vi "DFD Classical Design.vi"(5 "design method":T3(ring)=enum."Elliptic", 6 "fs [Hz]":dbl=1.0 format="%.2f", 7 "filter type":T10(ring), 8 "error in (no error)":errorcluster, 9 "ripple specs":T1={"passband"=0.1, "stopband"=60.0, "dB/linear? (T: dB)"=TRUE}, 10 "freq specs [Hz]":T2={"fpass 1"=0.2, "fstop 1"=0.3, "fpass 2 "=0.0, "fstop 2"=0.0}) -> (0 "error out":errorcluster, 2 "order":i32, 3 "filter out":T4={"mSRate_Fs"=1.0, "mSRate_Version"="2.0", "mSRate_Comments"="", "mSRate_OrgCoef"={"type"=enum."Undefined", "gain"=1.0, "coef a (k)"=[], "coef b (v)"=[]}, "mSRate_CurCoef"={"type"=enum."Undefined", "gain"=1.0, "coef a (k)"=[], "coef b (v)"=[]}, "mSRate_Quantized?"=FALSE, "mSRate_QCoef"={"type"=enum."Undefined", "gain"=1.0, "coef a (k)"=[], "coef b (v)"=[]}, "mSRate_QSettings"=[], "mSRate_Order"=0, "mSRate_Scaling"={"mSRate_ScaleByPowerOf2?"=FALSE, "mSRate_ScaleType"=enum."No Norm"}} {"mSRate_QSettings"."source" items=["Coef a/k"=0, "Coef b/v"=7, "Input"=1, "Output"=2, "Multiplicand"=3, "Product"=4, "Sum"=5, "Delay"=6, "Gain"=8]})   [LabVIEW 2017, in "NI_DigFilterLicensed.lvlib"]
doc: "Creates a lowpass, highpass, bandpass, or bandstop filter."
uses:
  <vilib>/addons/Digital Filter Design/NI_DigFilterLicensed.lvlib
  <vilib>/addons/Digital Filter Design/_Objects.llb/DFD Filter Obj.ctl
  <vilib>/addons/Digital Filter Design/_Objects.llb/DFD Filter Coef.ctl
  <vilib>/addons/Digital Filter Design/_Objects.llb/DFD Filter Structure Type Selector.ctl
  <vilib>/addons/Digital Filter Design/_Objects.llb/dfd_Internal Quantization Settings.ctl
  <vilib>/addons/Digital Filter Design/_Objects.llb/dfd_Internal Quantization Srcs.ctl
  <vilib>/addons/Digital Filter Design/_Objects.llb/DFD Coef Norm Type.ctl
  <vilib>/addons/Digital Filter Design/_Objects.llb/DFD Filter Frequence Specification (Design).ctl
  <vilib>/addons/Digital Filter Design/_Objects.llb/DFD Filter Ripple Specification (Design).ctl
  <vilib>/addons/Digital Filter Design/_REMEZ.llb/remez_fir filter type.ctl
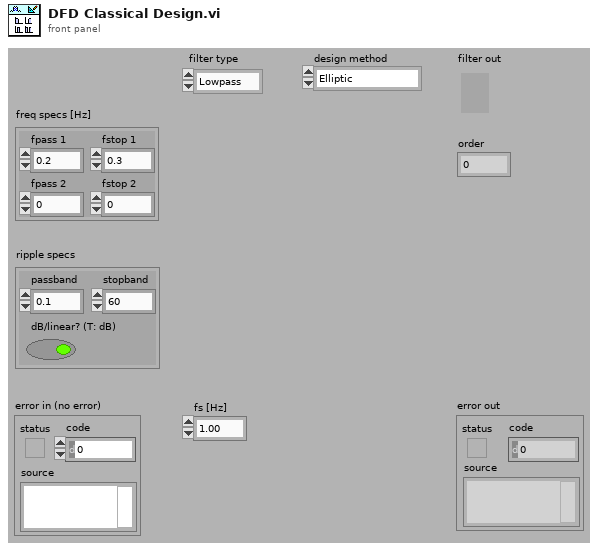
[diagram p1: front panel]
types:
  T1 = typedef "NI_DigFilterLicensed.lvlib/DFD Filter Ripple Specification (Design).ctl" = cluster{"passband":dbl, "stopband":dbl, "dB/linear? (T: dB)":bool}
  T2 = typedef "NI_DigFilterLicensed.lvlib/DFD Filter Frequence Specification (Design).ctl" = cluster{"fpass 1":dbl, "fstop 1":dbl, "fpass 2 ":dbl, "fstop 2":dbl}
  T3 = enum16{"Butterworth", "Chebyshev", "Inverse Chebyshev", "Elliptic", "Kaiser Window", "Dolph-Chebyshev Window", "Equi-Ripple FIR"}
  T4 = typedef "NI_DigFilterLicensed.lvlib/DFD Filter Obj.ctl" = cluster{"mSRate_Fs":dbl, "mSRate_Version":string, "mSRate_Comments":string, "mSRate_OrgCoef":T5, "mSRate_CurCoef":T5, "mSRate_Quantized?":bool, "mSRate_QCoef":T5, "mSRate_QSettings":T7[], "mSRate_Order":i32, "mSRate_Scaling":cluster{"mSRate_ScaleByPowerOf2?":bool, "mSRate_ScaleType":T9}}
  T5 = typedef "NI_DigFilterLicensed.lvlib/DFD Filter Coef.ctl" = cluster{"type":T6, "gain":dbl, "coef a (k)":dbl[], "coef b (v)":dbl[]}
  T6 = typedef "NI_DigFilterLicensed.lvlib/DFD Filter Structure Type Selector.ctl" = enum16{"Undefined", "FIR Direct Form", "FIR Direct Form Transposed", "FIR Symmetric", "FIR Antisymmetric", "IIR Direct Form I", "IIR Direct Form I Transposed", "IIR Direct Form II", "IIR Direct Form II Transposed", "IIR Cascaded Second Order Sections Form I", "IIR Cascaded Second Order Sections Form I Transposed", "IIR Cascaded Second Order Sections Form II", "IIR Cascaded Second Order Sections Form II Transposed", "Lattice Allpass (basic sections)", "Lattice Allpass (one multiplier sections)", "Lattice Allpass (normalized sections)", "Lattice AR (basic sections)", "Lattice AR (one multiplier sections)", "Lattice AR (normalized sections)", "Lattice MA (minimum phase)", "Lattice MA (maximum phase)", "Lattice ARMA (basic sections)", "Lattice ARMA (one multiplier sections)", "Lattice ARMA (normalized sections)"}
  T7 = typedef "NI_DigFilterLicensed.lvlib/dfd_Internal Quantization Settings.ctl" = cluster{"source":T8, "wl":i16, "iwl":i16, "overflow mode":enum16{"Saturation", "Wrap"}, "rounding mode":enum16{"Nearest", "Truncation"}, "signed?":bool}
  T8 = typedef "NI_DigFilterLicensed.lvlib/dfd_Internal Quantization Srcs.ctl" = u16
  T9 = typedef "NI_DigFilterLicensed.lvlib/DFD Coef Norm Type.ctl" = enum16{"No Norm", "Time Domain 1-Norm", "Time Domain 2-Norm", "Time Domain Inf-Norm"}
  T10 = enum16{"Lowpass", "Highpass", "Bandpass", "Bandstop"}
  T11 = typedef "NI_DigFilterLicensed.lvlib/remez_fir filter type.ctl" = enum32{"Symmetric", "Antisymmetric", "Differentiator", "Hilbert", "Minimum Phase", "Maximum Phase"}
  T12 = cluster{"passband ripple":dbl, "stopband atten":dbl}
  T13 = typedef "NI_DigFilterLicensed.lvlib/DFD Adv Band Spec.ctl" = cluster{"band specification":cluster{"freq":dbl, "amplitude":dbl, "weight":dbl}[], "ripple constraint":dbl}
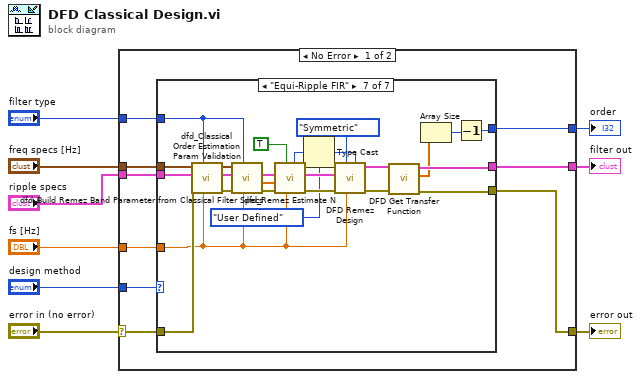
[diagram p0: block diagram]
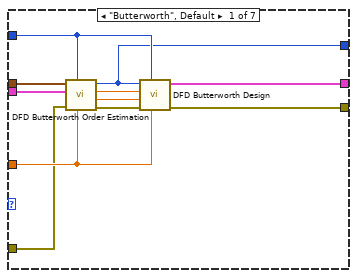
[diagram p2: hidden frame]
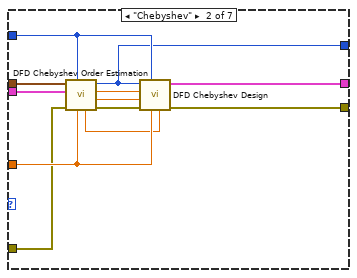
[diagram p3: hidden frame]
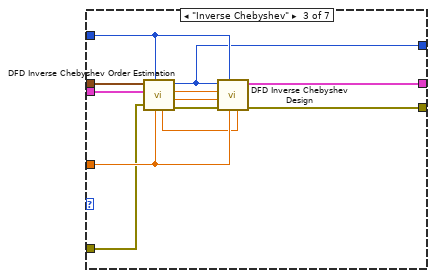
[diagram p4: hidden frame]
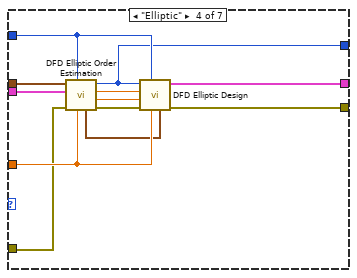
[diagram p5: hidden frame]
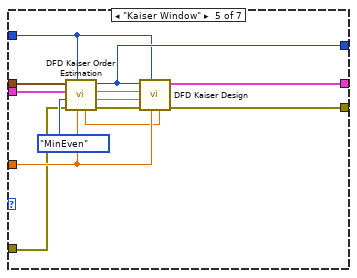
[diagram p6: hidden frame]
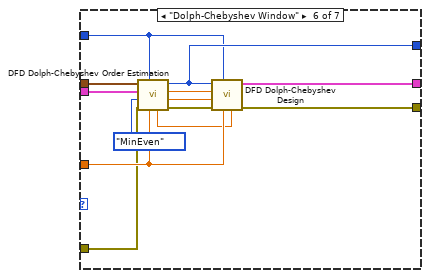
[diagram p7: hidden frame]
diagram:
  n1 = case shown="No Error" "error in (no error)" {
    selector: "error in (no error)" -> [w13 w118]
    tunnel: [w11 w118] -> w8
    tunnel: "design method" -> [w18 _]
    tunnel: "fs [Hz]" -> [w12 _]
    tunnel: "filter type" -> [w17 _]
    tunnel: [w10 _] -> w4
    tunnel: [w16 _] -> w3
    tunnel: "freq specs [Hz]" -> [w15 _]
    tunnel: "ripple specs" -> [w14 _]
    frame No Error {
      n2 = case shown="\"Equi-Ripple FIR\"" w18 {
        tunnel: w12 -> [w24 w36 w46 w60 w73 w87 w94]
        tunnel: w17 -> [w29 w39 w49 w65 w74 w88 w100]
        tunnel: [w28 w38 w52 w62 w71 w85 w113] -> w10
        tunnel: [w25 w37 w50 w63 w72 w86 w114] -> w11
        tunnel: [w26 w35 w47 w61 w75 w89 w110] -> w16
        tunnel: w15 -> [w23 w34 w45 w59 w69 w83 w101]
        tunnel: w14 -> [w22 w33 w44 w58 w68 w82 w97]
        tunnel: w13 -> [w21 w32 w43 w57 w67 w81 w96]
        frame "Butterworth", Default {
          n3 = call <vilib>:"DFD Butterworth Order Estimation.vi"("fs [Hz]"=w24, "filter type"=w29, "error in (no error)"=w21, "ripple specs"=w22, "freq specs [Hz]"=w23) -> ("error out"=w27:errorcluster, "low cutoff freq [Hz]"=w19:dbl, "high cutoff freq [Hz]"=w20:dbl, "estimated order"=w26:i32)  [unwired: 3 out]
          n4 = call <vilib>:"DFD Butterworth Design.vi"("fs [Hz]"=w24, "filter type"=w29, "error in (no error)"=w27, "low cutoff freq [Hz]"=w19, "high cutoff freq [Hz]"=w20, "order"=w26) -> ("error out"=w25:errorcluster, "filter out"=w28:T4)  [unwired: 4 out]
        }
        frame "Chebyshev" {
          n5 = call <vilib>:"DFD Chebyshev Order Estimation.vi"("fs [Hz]"=w36, "filter type"=w39, "error in (no error)"=w32, "ripple specs"=w33, "freq specs [Hz]"=w34) -> ("error out"=w40:errorcluster, "low cutoff freq [Hz]"=w31:dbl, "high cutoff freq [Hz]"=w41:dbl, "estimated order"=w35:i32, "passband ripple [dB]"=w30:dbl)  [unwired: 2 out]
          n6 = call <vilib>:"DFD Chebyshev Design.vi"("passband ripple [dB]"=w30, "fs [Hz]"=w36, "filter type"=w39, "error in (no error)"=w40, "low cutoff freq [Hz]"=w31, "high cutoff freq [Hz]"=w41, "order"=w35) -> ("error out"=w37:errorcluster, "filter out"=w38:T4)  [unwired: 3 out]
        }
        frame "Inverse Chebyshev" {
          n7 = call <vilib>:"DFD Inverse Chebyshev Order Estimation.vi"("fs [Hz]"=w46, "filter type"=w49, "error in (no error)"=w43, "ripple specs"=w44, "freq specs [Hz]"=w45) -> ("error out"=w51:errorcluster, "low cutoff freq [Hz]"=w48:dbl, "high cutoff freq [Hz]"=w53:dbl, "estimated order"=w47:i32, "stopband atten [dB]"=w42:dbl)  [unwired: 2 out]
          n8 = call <vilib>:"DFD Inverse Chebyshev Design.vi"("stopband atten [dB]"=w42, "fs [Hz]"=w46, "filter type"=w49, "error in (no error)"=w51, "low cutoff freq [Hz]"=w48, "high cutoff freq [Hz]"=w53, "order"=w47) -> ("error out"=w50:errorcluster, "filter out"=w52:T4)  [unwired: 3 out]
        }
        frame "Elliptic" {
          n9 = call <vilib>:"DFD Elliptic Order Estimation.vi"("fs [Hz]"=w60, "filter type"=w65, "error in (no error)"=w57, "ripple specs"=w58, "freq specs [Hz]"=w59) -> ("error out"=w64:errorcluster, "low cutoff freq [Hz]"=w55:dbl, "high cutoff freq [Hz]"=w56:dbl, "estimated order"=w61:i32, "ripples [dB]"=w54:T12)  [unwired: 2 out]
          n10 = call <vilib>:"DFD Elliptic Design.vi"("ripples [dB]"=w54, "fs [Hz]"=w60, "filter type"=w65, "error in (no error)"=w64, "low cutoff freq [Hz]"=w55, "high cutoff freq [Hz]"=w56, "order"=w61) -> ("error out"=w63:errorcluster, "filter out"=w62:T4)  [unwired: 3 out]
        }
        frame "Kaiser Window" {
          n11 = call <vilib>:"DFD Kaiser Order Estimation.vi"("fs [Hz]"=w73, "filter type"=w74, "error in (no error)"=w67, "order option"=enum16{"MinNum", "MinEven", "MinOdd"}."MinEven", "ripple specs"=w68, "freq specs [Hz]"=w69) -> ("error out"=w78:errorcluster, "low cutoff freq [Hz]"=w76:dbl, "high cutoff freq [Hz]"=w77:dbl, "estimated order"=w75:i32, "beta"=w66:dbl)  [unwired: 1 out]
          n12 = call <vilib>:"DFD Kaiser Design.vi"("beta"=w66, "fs [Hz]"=w73, "filter type"=w74, "error in (no error)"=w78, "low cutoff freq [Hz]"=w76, "high cutoff freq [Hz]"=w77, "order"=w75) -> ("error out"=w72:errorcluster, "filter out"=w71:T4)  [unwired: 3 out]
        }
        frame "Dolph-Chebyshev Window" {
          n13 = call <vilib>:"DFD Dolph-Chebyshev Order Estimation.vi"("fs [Hz]"=w87, "filter type"=w88, "error in (no error)"=w81, "order option"=enum16{"MinNum", "MinEven", "MinOdd"}."MinEven", "ripple specs"=w82, "freq specs [Hz]"=w83) -> ("error out"=w91:errorcluster, "low cutoff freq [Hz]"=w90:dbl, "high cutoff freq [Hz]"=w80:dbl, "estimated order"=w89:i32, "ripple ratio [dB]"=w79:dbl)  [unwired: 1 out]
          n14 = call <vilib>:"DFD Dolph-Chebyshev Design.vi"("ripple ratio [dB]"=w79, "fs [Hz]"=w87, "filter type"=w88, "error in (no error)"=w91, "low cutoff freq [Hz]"=w90, "high cutoff freq [Hz]"=w80, "order"=w89) -> ("error out"=w86:errorcluster, "filter out"=w85:T4)  [unwired: 3 out]
        }
        frame "Equi-Ripple FIR" {
          n15 = call <vilib>:"dfd_Classical Order Estimation Param Validation.vi"("fs [Hz]"=w94, "filter type"=w100, "error in (no error)"=w96, "ripple specs"=w97, "freq specs [Hz]"=w101) -> ("error out"=w95:errorcluster, "dup ripple specs"=w98:T1, "dup freq specs [Hz]"=w99:T2)  [unwired: 1 in, 3 out]
          n16 = call <vilib>:"dfd_Build Remez Band Parameter from Classical Filter Specs.vi"("fs [Hz]"=w94, "filter type"=w100, "error in (no error)"=w95, "ripple specs"=w98, "freq specs [Hz]"=w99) -> ("error out"=w108:errorcluster, "band ripples"=w107:dbl[], "band parameters"=w103:T13[])  [unwired: 1 in, 3 out]
          n17 = call <vilib>:"dfd_Remez Estimate N.vi"("fs [Hz]"=w94, "auto order"=TRUE ("set constrain"), "error in (no error)"=w108, "band ripple"=w107, "band parameters"=w103) -> ("error out"=w109:errorcluster, "band parameters dup"=w105:T13[], "estimated order"=w106:i32, "minimum order"=w104:enum32{"user defined", "minEven", "minOdd"})  [unwired: 3 out]
          n18 = Type Cast(type=enum32{"User Defined", "MinEven", "MinOdd"}."User Defined" ("minimum order"), x=w104) -> (*(type *) &x=w93:enum32{"User Defined", "MinEven", "MinOdd"})
          n19 = call <vilib>:"DFD Remez Design.vi"("minimum order"=w93, "fs [Hz]"=w94, "filter type"=remez_fir_filter_type."Symmetric", "error in (no error)"=w109, "band specs"=w105, "order"=w106) -> ("error out"=w115:errorcluster, "filter out"=w116:T4)  [unwired: 1 in, 3 out]
          n20 = call <vilib>:"DFD Get Transfer Function.vi"("error in (no error)"=w115, "filter in"=w116) -> ("error out"=w114:errorcluster, "numerator"=w112:dbl[], "filter out"=w113:T4)  [unwired: 7 out]
          n21 = Array Size(array=w112) -> (size(s)=w111:i32)
          n22 = Decrement(x=w111) -> (x-1=w110:i32)
        }
      }
    }
    frame Error {
    }
  }
  "error out" <- w8
  "filter out" <- w4
  "order" <- w3
